vi "Test Flip ARGB.vi"(8 "error in (no error)":errorcluster, 11 "Test Case In":refnum<class "01_Image.lvclass">) -> (0 "error out":errorcluster, 3 "Test Case Out":refnum<class "01_Image.lvclass">)   [LabVIEW 2020, in "test.lvlib" / "01_Image.lvclass"]
uses:
  01_Image.lvclass
  C:/Program Files (x86)/National Instruments/LabVIEW 2026/vi.lib/Astemes/LUnit/Test Case.lvclass
  common/Image Size (Integer).ctl
  <vilib>/Astemes/LUnit/Test Case.lvclass/Test Case.ctl
  image/New Image (ARGB Preallocated).vi
  image/Flip (ARGB Y-Axis).vi
  4993e8ee-a06a-463a-9684-69129f64d5ce.vi
  image/Copy Array to Image.vi
  image/Copy Array to Image (ARGB).vi
  image/New Image (ARGB Preallocated).vi/3321fa97-f432-4e1e-8db9-a0df79aed21b.vi
  image/ARGB Colour to U32 Pixel Value.vi
  image/Flip (ARGB Y-Axis).vi/348de330-10c9-445f-8d54-7780e9118077.vi
  <vilib>/Astemes/LUnit/Core/LUnit Test Case/Private/Append Pass Result.vi
  <vilib>/Astemes/LUnit/Core/LUnit Test Case/Private/Append Fail Result.vi
  4993e8ee-a06a-463a-9684-69129f64d5ce.vi/9c5d11cd-9439-4240-a1ee-d9baace9c924.vi
  <vilib>/Astemes/LUnit/Core/LUnit Test Case/Private/Run In UI.vi
  <vilib>/Utility/error.llb/Clear Errors.vi
  <vilib>/Utility/error.llb/Error Cluster From Error Code.vi
  <vilib>/picture/pixmap.llb/Flatten Pixmap.vi
  image/image.lvlib
  common/common.lvlib
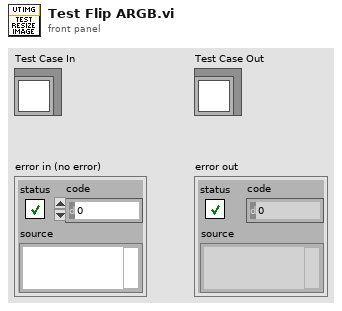
[diagram p1: front panel]
types:
  T1 = typedef "common.lvlib/Image Size (Integer).ctl" = cluster{"Width":u16, "Height":u16}
  T2 = typedef "image.lvlib/ARGB Image.ctl" = refnum<data-value>
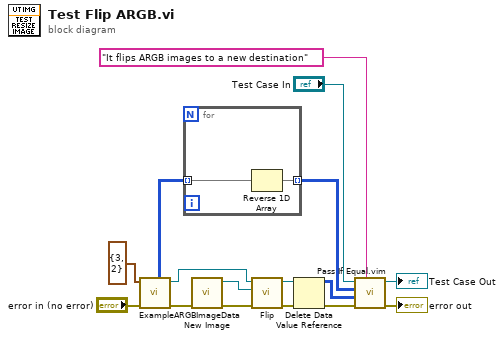
[diagram p0: block diagram]
diagram:
  n1 = call "ExampleARGBImageData.vi"("error in (no error)"="error in (no error)", "Image Size"=T1 {"Width"=3, "Height"=2}) -> ("error out"=w5:errorcluster, "Data Value Reference out"=w3:T2, "ARGB Array Data"=w1:u32[][])  [unwired: 6 in, 1 out]
  n2 = for {
    tunnel: [w18] -> w6 mode=indexing
    tunnel: w1 -> [w17] mode=indexing
    n3 = Reverse 1D Array(array=w17) -> (reversed array=w18:u32[])
  }
  n4 = call-poly "New Image.vi"("error in (no error)"=w5) -> ("error out"=w9:errorcluster, "ARGB Image"=w7:T2)  [unwired: 9 in]
  n5 = call-poly "Flip.vi"("error in (no error)"=w9, "ARGB Destination Image in"=w7, "ARGB Source Image in"=w3) -> ("error out"=w10:errorcluster, "ARGB  Destination Image"=w11:T2)  [unwired: 7 in]
  n6 = Delete Data Value Reference(data value reference=w11, error in=w10) -> (data value=w8:u32[][], error out=w13:errorcluster)
  n7 = call "Pass If Equal.vim"("Description"="It flips ARGB images to a new destination", "error in (no error)"=w13, "Actual"=w8, "Expected"=w6, "LUnit Test Case In"="Test Case In") -> ("error out"=→"error out":errorcluster, "LUnit Test Case Out"=→"Test Case Out":refnum<class "01_Image.lvclass">)  [unwired: 5 in]
